vi "oa_Full Spectrum Transform.vi"(6 "direction":u16(ring)=1 items=["CCW", "CW"], 9 "Phase Lag (X-Y in radians)":dbl[](array[numeric]), 10 "Y Magnitude":dbl[](array[numeric]), 11 "X Magnitude":dbl[](array[numeric])) -> (2 "Reverse Precession Magnitude":dbl[](array[numeric]), 3 "Forward Precession Magnitude":dbl[](array[numeric]))   [LabVIEW 2017]
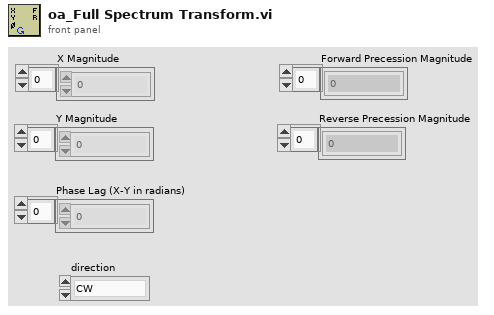
[diagram p1: front panel]
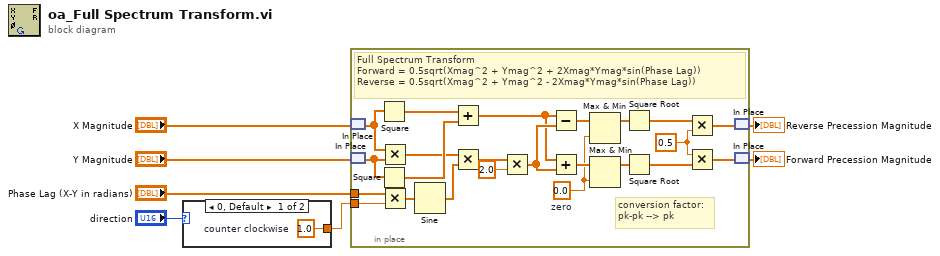
[diagram p0: block diagram]
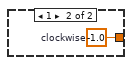
[diagram p2: hidden frame]
diagram:
  n1 = case shown="0, Default" "direction" {
    tunnel: [w8 w9] -> w6
    frame 0, Default {
      w8 = 1.0  # counter clockwise
    }
    frame 1 {
      w9 = -1.0  # clockwise
    }
  }
  n2 = in-place {
    in-place-border: "Phase Lag (X-Y in radians)" -> [w32]
    in-place-border: w6 -> [w31]
    w10 = 0.5 ("amplitude")
    w15 = 0.0  # zero
    # "conversion factor:\npk-pk --> pk"
    # "Full Spectrum Transform\nForward = 0.5sqrt(Xmag^2 + Ymag^2 + 2Xmag*Ymag*sin(Phase Lag))\nReverse = 0.5sqrt(Xmag^2 + Ymag^2 - 2Xmag*Ymag*sin(Phase Lag))"
    n3 = in-place-match #1("X Magnitude") -> (w21:dbl[])
    n4 = in-place-match #2("Y Magnitude") -> (w20:dbl[])
    n5 = Square(x=w21) -> (x^2=w26:dbl[])
    n6 = Square(x=w20) -> (x^2=w27:dbl[])
    n7 = Multiply(x=w21, y=w20) -> (x*y=w22:dbl[])
    n8 = Multiply(x=w32, y=w31) -> (x*y=w30:dbl[])
    n9 = Sine(x=w30) -> (sin(x)=w23:dbl[])
    n10 = Add(x=w26, y=w27) -> (x+y=w28:dbl[])
    n11 = Multiply(x=w22, y=w23) -> (x*y=w24:dbl[])
    n12 = Multiply(x=w24, y=2.0 ("amplitude")) -> (x*y=w29:dbl[])
    n13 = Subtract(x=w28, y=w29) -> (x-y=w19:dbl[])
    n14 = Add(x=w28, y=w29) -> (x+y=w18:dbl[])
    n15 = Max & Min(x=w19, y=w15) -> (max(x,y)=w17:dbl[])  [unwired: 1 out]
    n16 = Max & Min(x=w18, y=w15) -> (max(x,y)=w16:dbl[])  [unwired: 1 out]
    n17 = Square Root(x=w17) -> (sqrt(x)=w12:dbl[])
    n18 = Square Root(x=w16) -> (sqrt(x)=w14:dbl[])
    n19 = Multiply(x=w12, y=w10) -> (x*y=w11:dbl[])
    n20 = Multiply(x=w10, y=w14) -> (x*y=w13:dbl[])
    n21 = in-place-match #1(w11) -> (→"Reverse Precession Magnitude":dbl[])
    n22 = in-place-match #2(w13) -> (→"Forward Precession Magnitude":dbl[])
  }
